vi "Read Current Leakage Threshold.vi"(0 "VISA resource name":refnum<visa-resource-name>, 1 "Source Current Limit (1 A)":dbl=1.0, 2 "Source Delay (0.3 S)":dbl=0.3, 3 "Wait Time (1 S)":dbl=1.0, 5 "Source Measure Unit Channel (0: Channel A)":i32(ring) items=["Channel A", "Channel B"], 7 "Voltage Level (0 V)":dbl, 9 "Threshold (1E-6 A)":dbl=1e-06, 11 "error in (no error)":errorcluster, 12 "Measure Current Limit (1E-5 A)":dbl=1e-05, 13 "Measure Delay (0.1 S)":dbl=0.1) -> (4 "VISA resource name out":refnum<visa-resource-name>, 6 "Compared Result":bool, 15 "error out":errorcluster)   [LabVIEW 2019, in "Keithley 2600 Series.lvlib"]
doc: "Performs a current leakage measurement compares it to a threshold."
uses:
  Keithley 2600 Series.lvlib
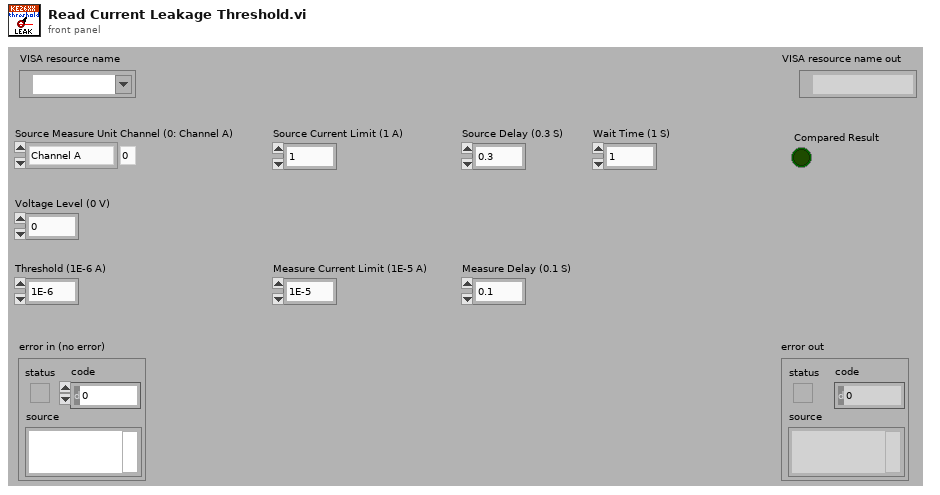
[diagram p1: front panel]
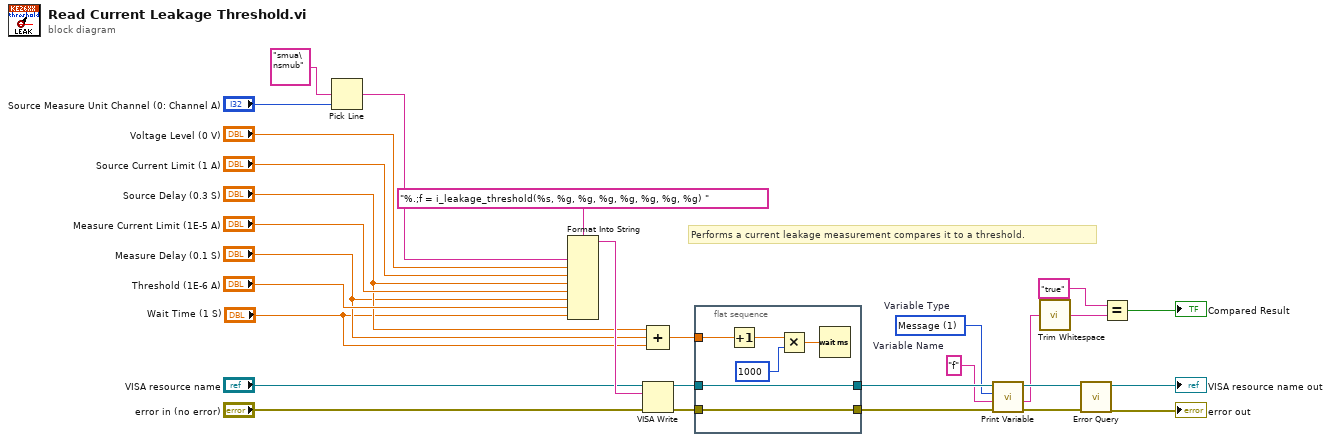
[diagram p0: block diagram]
diagram:
  w2 = "f"  # Variable Name
  w3 = 1 items=["Number", "Message"]  # Variable Type
  # "Performs a current leakage measurement compares it to a threshold."
  n1 = Pick Line(multi-line string="smua\nsmub", line index="Source Measure Unit Channel (0: Channel A)") -> (output string=w17:string)  [unwired: 1 in]
  n2 = Format Into String(format string="%.;f = i_leakage_threshold(%s, %g, %g, %g, %g, %g, %g, %g) ", w17, "Voltage Level (0 V)", "Source Current Limit (1 A)", "Source Delay (0.3 S)", "Measure Current Limit (1E-5 A)", "Measure Delay (0.1 S)", "Threshold (1E-6 A)", "Wait Time (1 S)") -> (resulting string=w24:string)  [unwired: 2 in, 1 out]
  n3 = VISA Write(VISA resource name="VISA resource name", write buffer=w24, error in (no error)="error in (no error)") -> (VISA resource name out=w14:refnum<visa-resource-name>, error out=w13:errorcluster)  [unwired: 1 out]
  n4 = Compound Arithmetic op=ADD("Source Delay (0.3 S)", "Measure Delay (0.1 S)", "Wait Time (1 S)") -> (w9:dbl)
  n5 = flat-sequence {
    tunnel: w14 -> [w35]
    tunnel: w13 -> [w34]
    tunnel: [w35] -> w8
    tunnel: [w34] -> w7
    tunnel: w9 -> [w31]
    frame #0 {
      n6 = Increment(x=w31) -> (x+1=w30:dbl)
      n7 = Multiply(x=w30, y=1000) -> (x*y=w32:dbl)
      n8 = Wait (ms)(milliseconds to wait=w32) -> ()  [unwired: 1 out]
    }
  }
  n9 = call "Print Variable.vi"("error in (no error)"=w7, "Variable Name"=w2, "Variable Type (0: Number)"=w3, "VISA resource name"=w8) -> ("error out"=w5:errorcluster, "Message"=w4:string, "VISA resource name out"=w6:refnum<visa-resource-name>)  [unwired: 4 in, 1 out]
  n10 = call <vilib>:"Trim Whitespace.vi"("string"=w4) -> ("trimmed string"=w16:string)  [unwired: 1 in]
  n11 = call "Error Query.vi"("error in (no error)"=w5, "VISA resource name"=w6) -> ("error out"=→"error out":errorcluster, "VISA resource name out"=→"VISA resource name out":refnum<visa-resource-name>)  [unwired: 6 in, 2 out]
  n12 = Equal?(x="true", y=w16) -> (x = y?=→"Compared Result":bool)
